vi "destroy.vi"(8 "error in (no error)":errorcluster, 11 "simple_html_chat_ui in":refnum<class "simple_html_chat_ui.lvclass">) -> (0 "error out":errorcluster, 3 "simple_html_chat_ui out":refnum<class "simple_html_chat_ui.lvclass">)   [LabVIEW 2020, in "simple_html_chat_ui.lvclass"]
uses:
  simple_html_chat_ui.lvclass
  utils/ui_user_event.ctl
  simple_html_chat_ui.lvclass/simple_html_chat_ui.ctl
  <vilib>/httpClient/POSTBuffer.vi
  <vilib>/httpClient/LabVIEWHTTPClient.lvlib
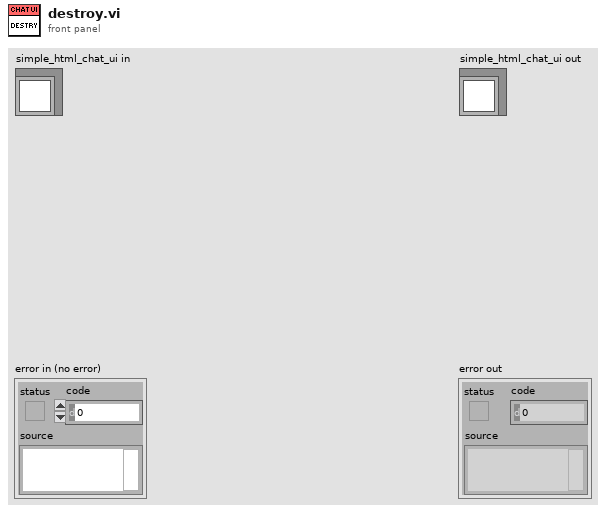
[diagram p1: front panel]
types:
  T1 = typedef "ui_user_event.ctl" = enum16{"Initialize", "Generate", "Get Reference", "Destroy"}
  T2 = typedef "LabVIEWHTTPClient.lvlib/ClientHandle.ctl" = refnum<k1>
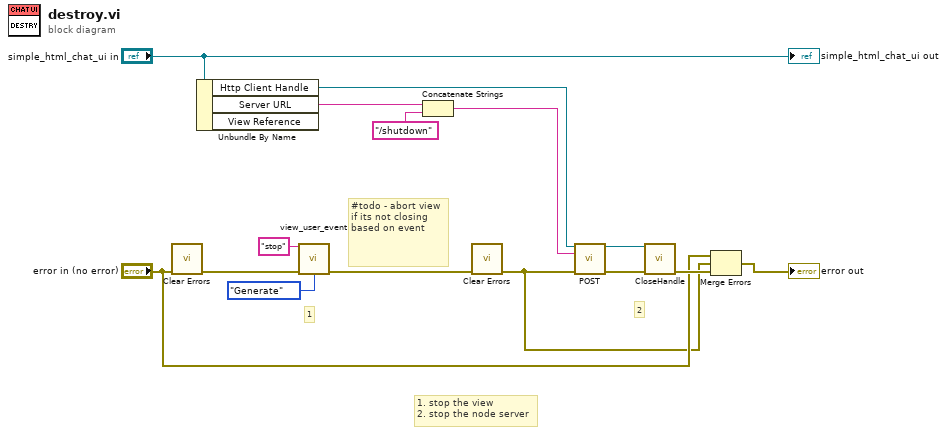
[diagram p0: block diagram]
diagram:
  # "#todo - abort view if its not closing based on event"
  # "2"
  # "1"
  # "1. stop the view\n2. stop the node server"
  n1 = call <vilib>:"Clear Errors.vi"("error in (no error)"="error in (no error)") -> ("error out"=w4:errorcluster)  [unwired: 5 in, 1 out]
  n2 = Unbundle By Name("simple_html_chat_ui in") -> ("Http Client Handle"=w11:T2, "Server URL"=w10:string)  [unwired: 1 out]
  n3 = call "view_user_event.vi"("State"="stop", "error in (no error)"=w4, "Operation"=ui_user_event."Generate") -> ("error out"=w7:errorcluster)  [unwired: 11 in, 1 out]
  n4 = Concatenate Strings(w10, "/shutdown" ("string")) -> (w8:string)
  n5 = call <vilib>:"Clear Errors.vi"("error in (no error)"=w7) -> ("error out"=w1:errorcluster)  [unwired: 5 in, 1 out]
  n6 = call-poly <vilib>:"POST.vi"("client handle"=w11, "url"=w8, "error in (no error)"=w1) -> ("client handle out"=w12:T2, "error out"=w13:errorcluster)  [unwired: 9 in, 2 out]
  n7 = call <vilib>:"CloseHandle.vi"("client handle"=w12, "error in (no error)"=w13) -> ("error out"=w15:errorcluster)  [unwired: 13 in]
  n8 = Merge Errors("error in (no error)", w1, w15) -> (→"error out":errorcluster)
  "simple_html_chat_ui out" <- "simple_html_chat_ui in"
